vi "In_S2F15.vi"(8 "error in (no error)":errorcluster, 11 "S2 Message Class in":refnum<class "S2 Message Class.lvclass">) -> (0 "error out":errorcluster, 1 "OK?":bool, 2 "S2F15":T1, 3 "S2 Message Class out":refnum<class "S2 Message Class.lvclass">)   [LabVIEW 2020, in "SECS Communication.lvlib" / "S2 Message Class.lvclass"]
uses:
  S2 Message Class.lvclass
  D:/Dropbox/SECS/SECS_GEM v1.0.6/Com/SECS Communication/SECS-II Class/SECS-II Class.lvclass
  S2F15.ctl
  SECS-II Class/Format Code.ctl
  SECS-II Class/SECS-II Class.lvclass/SECS-II Class.ctl
  SECS-II Class/Variant To Data_U4.vi
  SECS-II Class/SECS-II Class.lvclass
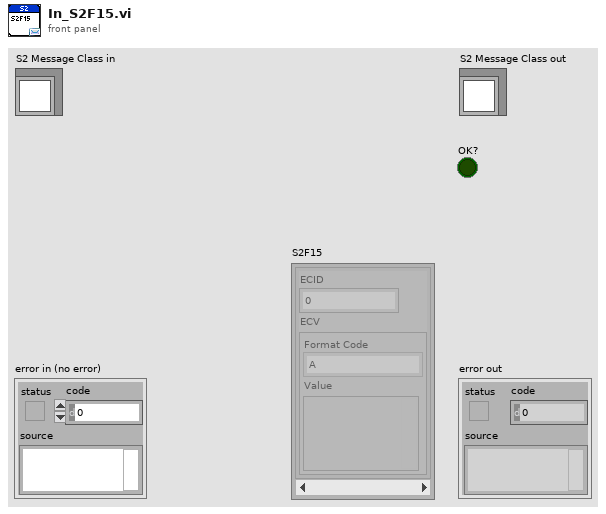
[diagram p1: front panel]
types:
  T1 = typedef "SECS Communication.lvlib/S2 Message Class.lvclass/S2F15.ctl" = cluster{"ECID":u32, "ECV":cluster{"Format Code":T2, "Value":variant}}[]
  T2 = typedef "SECS Communication.lvlib/SECS-II Class.lvclass/Format Code.ctl" = enum16{"L", "A", "B", "Boolean", "J", "I1", "I2", "I4", "I8", "U1", "U2", "U4", "U8", "F4", "F8", "Char"}
  T3 = typedef "SECS Communication.lvlib/SECS-II Class.lvclass/Message Data.ctl" = cluster{"Index":i32, "Data Item Format":T4, "Format Code":T2, "Parent Index":i32, "Child Index":i32[], "Data":variant}
  T4 = typedef "SECS Communication.lvlib/SECS-II Class.lvclass/Data Item Format.ctl" = enum16{"Data Type", "Value"}
  T5 = cluster{"Data":u32, cluster{"Format Code":T2, "Data":variant}}
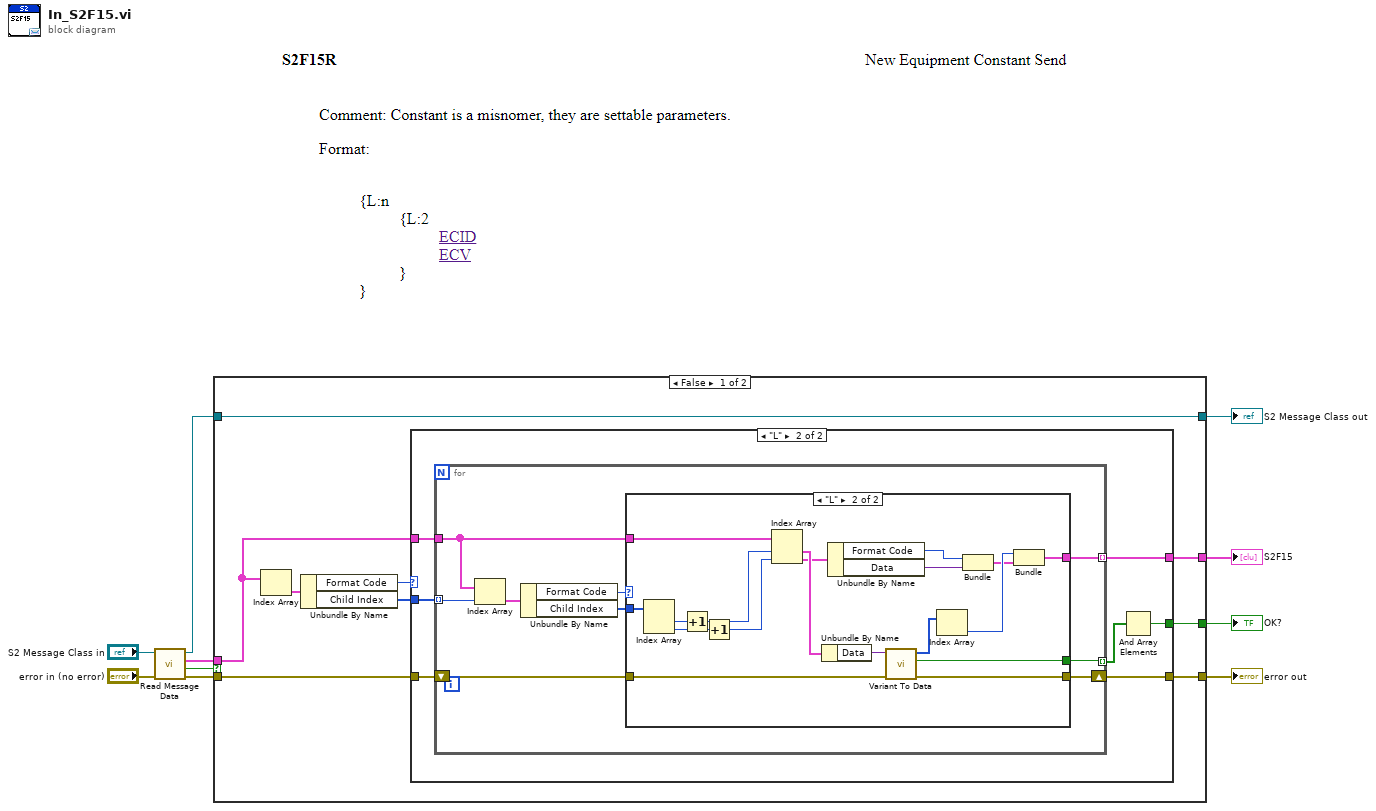
[diagram p0: block diagram]
diagram:
  n1 = call "Read Message Data.vi"("error in (no error)"="error in (no error)", "SECS-II Class in"="S2 Message Class in") -> ("error out"=w10:errorcluster, "Empty?"=w4:bool, "Message Data"=w9:T3[], "SECS-II Class out"=w3:refnum<class "S2 Message Class.lvclass">)  [unwired: 6 in]
  n2 = case shown="False" w4 {
    tunnel: w10 -> [w17 w56]
    tunnel: w9 -> [w16 _]
    tunnel: [w15 _] -> w6
    tunnel: [w14 w56] -> w5
    tunnel: w3 -> [w12 w57]
    tunnel: [w12 w57] -> w2
    tunnel: [w11 _] -> w1
    frame False {
      n3 = Index Array(array=w16) -> (element=w19:T3)  [unwired: 1 in]
      n4 = Unbundle By Name(w19) -> ("Format Code"=w13:T2, "Child Index"=w18:i32[])
      n5 = case shown="\"L\"" w13 {
        tunnel: w18 -> [_ w27]
        tunnel: w17 -> [w20 w26]
        tunnel: w16 -> [_ w25]
        tunnel: [_ w24] -> w15
        tunnel: [w20 w23] -> w14
        tunnel: [_ w21] -> w11
        frame Default {
        }
        frame "L" {
          n6 = for {
            tunnel: w27 -> [w35] mode=indexing
            tunnel: w25 -> [w33]
            shift-right: [w31] -> w23
            shift-left: w26 -> [w32]
            tunnel: [w30] -> w24 mode=indexing
            tunnel: [w28] -> w22 mode=indexing
            n7 = Index Array(array=w33, index=w35) -> (element=w36:T3)
            n8 = Unbundle By Name(w36) -> ("Format Code"=w29:T2, "Child Index"=w34:i32[])
            n9 = case shown="\"L\"" w29 {
              tunnel: w34 -> [_ w55]
              tunnel: w33 -> [_ w54]
              tunnel: w32 -> [w37 w48]
              tunnel: [w37 w42] -> w31
              tunnel: [_ w39] -> w30
              tunnel: [_ w38] -> w28
              frame Default {
              }
              frame "L" {
                n10 = Index Array(array=w55) -> (element #1=w53:i32, element #2=w52:i32)  [unwired: 2 in]
                n11 = Increment(x=w53) -> (x+1=w51:i32)
                n12 = Increment(x=w52) -> (x+1=w50:i32)
                n13 = Index Array(array=w54, index #1=w51, index #2=w50) -> (element #1=w49:T3, element #2=w46:T3)
                n14 = Unbundle By Name(w49) -> ("Data"=w47:variant)
                n15 = Unbundle By Name(w46) -> ("Format Code"=w44:T2, "Data"=w45:variant)
                n16 = call-poly "Variant To Data.vi"("error in (no error)"=w48, "Variant"=w47) -> ("error out"=w42:errorcluster, "OK?"=w38:bool, "Data"=w43:u32[])  [unwired: 7 in]
                n17 = Index Array(array=w43) -> (element=w41:u32)  [unwired: 1 in]
                n18 = Bundle("Format Code"=w44, "Data"=w45) -> (w40:cluster{"Format Code":T2, "Data":variant})  [unwired: 1 in]
                n19 = Bundle("Data"=w41, w40) -> (w39:T5)  [unwired: 1 in]
              }
            }
          }
          n20 = And Array Elements(Boolean array=w22) -> (logical AND=w21:bool)
        }
      }
    }
    frame True {
    }
  }
  "error out" <- w5
  "S2 Message Class out" <- w2
  "S2F15" <- w6
  "OK?" <- w1
